vi "Write filepath.vi"(8 "error in (no error)":errorcluster, 10 "Filepath":path, 11 "CFitsIO in":refnum<class "CFitsIO.lvclass">) -> (0 "error out":errorcluster, 3 "CFitsIO out":refnum<class "CFitsIO.lvclass">)   [LabVIEW 2016, in "CFitsIO.lvclass"]
uses:
  CFitsIO.lvclass
  CFitsIO.lvclass/CFitsIO.ctl
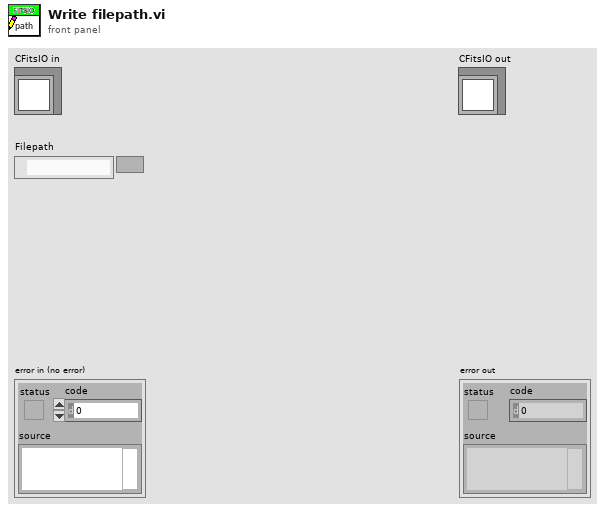
[diagram p1: front panel]
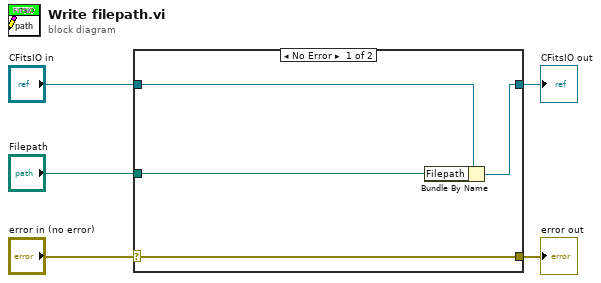
[diagram p0: block diagram]
diagram:
  n1 = case shown="No Error" "error in (no error)" {
    selector: "error in (no error)" -> [w9 w10]
    tunnel: [w9 w10] -> w4
    tunnel: [w7 w11] -> w2
    tunnel: "CFitsIO in" -> [w8 w11]
    tunnel: "Filepath" -> [w6 _]
    frame No Error {
      n2 = Bundle By Name(cluster=w8, "Filepath"=w6) -> (w7:refnum<class "CFitsIO.lvclass">)
    }
    frame Error {
    }
  }
  "error out" <- w4
  "CFitsIO out" <- w2
